vi "Get Instr Ident.vi"(8 "error in":errorcluster, 11 "CFG Base in":refnum<class "CFG Base.lvclass">) -> (0 "error out":errorcluster, 2 "Instr Ident":string, 3 "CFG Base out":refnum<class "CFG Base.lvclass">)   [LabVIEW 2024, in "HAL.lvlib" / "CFG Base.lvclass"]
uses:
  CFG Base.lvclass
  CFG Base.lvclass/CFG Base.ctl
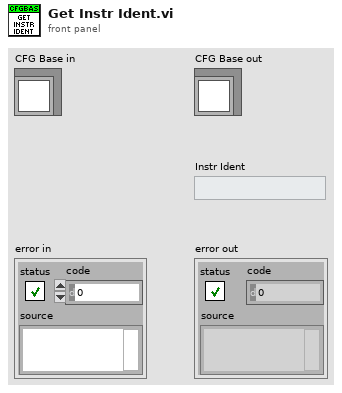
[diagram p1: front panel]
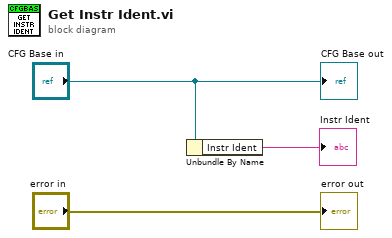
[diagram p0: block diagram]
diagram:
  n1 = Unbundle By Name("CFG Base in") -> ("Instr Ident"=→"Instr Ident":string)
  "error out" <- "error in"
  "CFG Base out" <- "CFG Base in"
